vi "ATSpectrograph_logEvent_reportedLinearStagePosition.vi"(8 "error in (no error)":errorcluster, 11 "logevent_reportedLinearStagePosition_Ctl":T1) -> (0 "error out":errorcluster, 2 "function return":i32, 3 "logevent_reportedLinearStagePosition_Ctl out":T1)   [LabVIEW 2016, in "SALLV_ATSpectrograph.lvlib"]
doc: "int ATSpectrograph_shm_logEvent_reportedLinearStagePositionLV(ATSpectrograph_logevent_reportedLinearStagePositionLV *logevent_reportedLinearStagePosition_Ctl );"
uses:
  SALLV_ATSpectrograph.lvlib
  DataTypes/logevent_reportedLinearStagePosition.ctl
  SALLV_ATSpectrograph.so
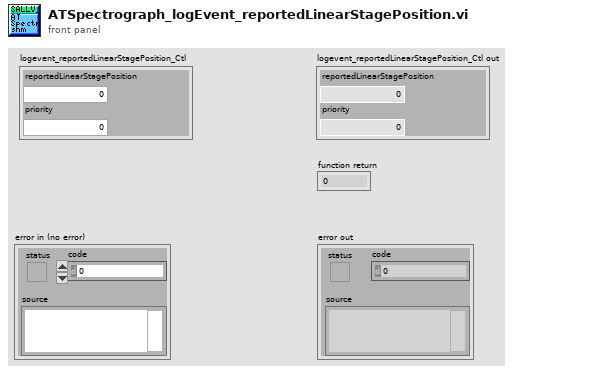
[diagram p1: front panel]
types:
  T1 = typedef "SALLV_ATSpectrograph.lvlib/logevent_reportedLinearStagePosition.ctl" = cluster{"reportedLinearStagePosition":sgl, "priority":i32}
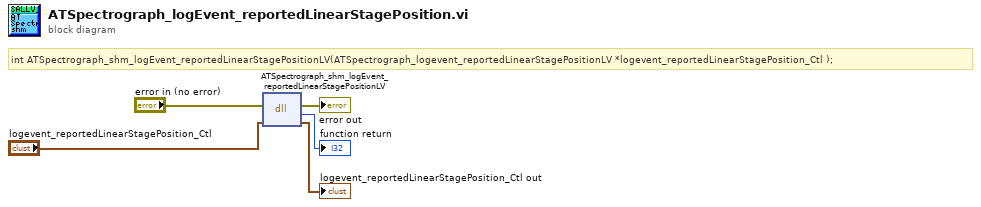
[diagram p0: block diagram]
diagram:
  # "int ATSpectrograph_shm_logEvent_reportedLinearStagePositionLV(ATSpectrograph_logevent_reportedLinearStagePositionLV *logevent_reportedLinearStagePosition_Ctl );"
  n1 = dll-call lib="home/harini/tcs/SALLV_ATSpectrograph/SALLV_ATSpectrograph.*" fn="ATSpectrograph_shm_logEvent_reportedLinearStagePositionLV"(error in="error in (no error)", "logevent_reportedLinearStagePosition_Ctl"="logevent_reportedLinearStagePosition_Ctl") -> (error out=→"error out":errorcluster, →"function return":i32, "logevent_reportedLinearStagePosition_Ctl"=→"logevent_reportedLinearStagePosition_Ctl out":T1)  [unwired: 2 in, 1 out]
